vi "Host - Get Remote IO Module Data.vi"(8 "error in (no error)":errorcluster, 11 "Remote IO Mod IOVs":refnum<k21>[](array[refnum])) -> (0 "error out":errorcluster, 3 "Modules":T1[](array[typedef]))   [LabVIEW 2019, in "SEECD System Explorer.lvlib"]
uses:
  SEECD System Explorer.lvlib
  Type Defs/Host - Module.ctl
  <resource>/objmgr/IndComECAT.rc
  Type Defs/IOV Container Contents.ctl
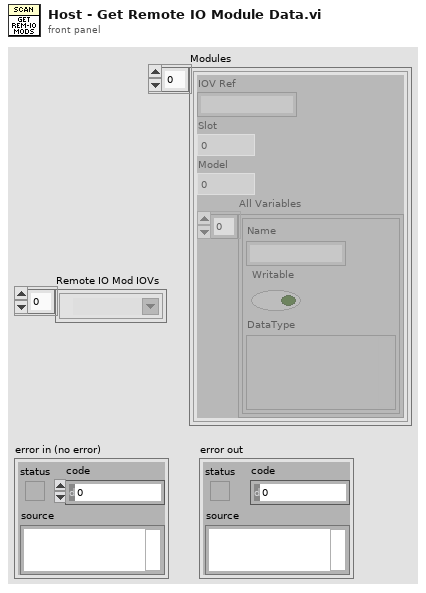
[diagram p1: front panel]
types:
  T1 = typedef "SEECD System Explorer.lvlib/Host - Module.ctl" = cluster{"IOV Ref":string, "Slot":u32, "Model":u32, "All Variables":T2[]}
  T2 = typedef "SEECD System Explorer.lvlib/IOV Container Contents.ctl" = cluster{"Name":string, "Writable":bool, "DataType":variant}
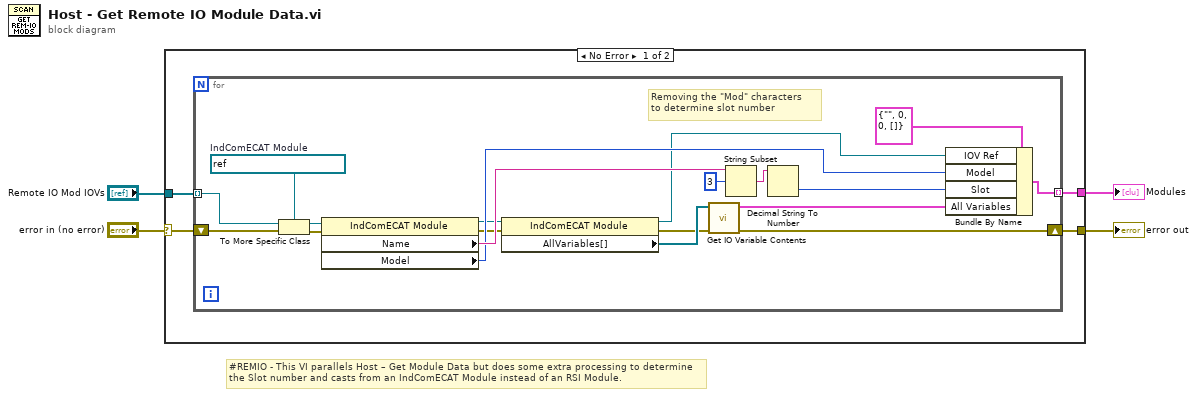
[diagram p0: block diagram]
diagram:
  # "#REMIO - This VI parallels Host – Get Module Data but does some extra processing to determine the Slot number and casts from an IndComECAT Module instead of an RSI Module."
  n1 = case shown="No Error" "error in (no error)" {
    selector: "error in (no error)" -> [w6 w28]
    tunnel: [w8 _] -> w4
    tunnel: [w7 w28] -> w3
    tunnel: "Remote IO Mod IOVs" -> [w5 _]
    frame No Error {
      n2 = for {
        shift-right: [w9] -> w7
        shift-left: w6 -> [w20]
        tunnel: [w27] -> w8 mode=indexing
        tunnel: w5 -> [w22] mode=indexing
        w21 = refnum<k21> refnum  # IndComECAT Module
        # "Removing the \"Mod\" characters\nto determine slot number"
        n3 = To More Specific Class(target class=w21, reference=w22, error in=w20) -> (specific class reference=w18:refnum<k21>, error out=w19:errorcluster)
        n4 = property class="IndComECAT Module"(reference=w18, error in=w19) -> (reference out=w14:refnum<k21>, error out=w15:errorcluster, "Name"=w25:string, "Model"=w16:u32)
        n5 = property class="IndComECAT Module"(reference=w14, error in=w15) -> (reference out=w11:refnum<k21>, error out=w12:errorcluster, "AllVariables[]"=w13:refnum<k21>[])
        n6 = call "Get IO Variable Contents.vi"("error in (no error)"=w12, "AllVariables[]"=w13) -> ("error out"=w9:errorcluster, "All Variables Contents"=w10:T2[])  [unwired: 8 in]
        n7 = String Subset(string=w25, offset (0)=3) -> (substring=w23:string)  [unwired: 1 in]
        n8 = Decimal String To Number(string=w23) -> (number=w17:i32)  [unwired: 2 in, 1 out]
        n9 = Bundle By Name(cluster=T1 {"IOV Ref"="", "Slot"=0, "Model"=0, "All Variables"=[]} ("Module"), "IOV Ref"=w11, "Model"=w16, "Slot"=w17, "All Variables"=w10) -> (w27:T1)
      }
    }
    frame Error {
    }
  }
  "Modules" <- w4
  "error out" <- w3
